vi "LoadTrafficLightsQueue with Exit.vi"(0 "Queue Ref in":refnum<queue>, 2 "Walk":bool) -> ()   [LabVIEW 2012]
doc: "Used to Enqueue the Walk Element when Walk button has been pressed. Uses a Queue Reference to efficiently read the address of Red State, Enqueues rest of elements and places Walk State at the front of the Queue.\nFor use alongside VI's that require the Exit Element."
uses:
  Controls/Traffic Light States (with Walk and Exit State).ctl
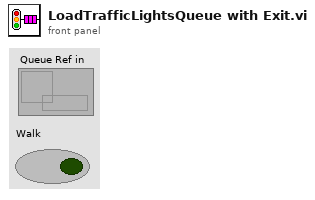
[diagram p1: front panel]
types:
  T1 = typedef "Traffic Light States (with Walk and Exit State).ctl" = enum16{"Red", "RedAmber", "Green", "Amber", "Walk", "Exit"}
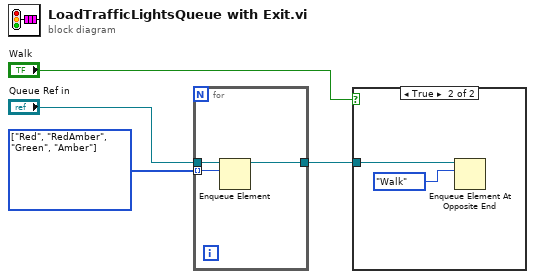
[diagram p0: block diagram]
diagram:
  w1 = T1[] [enum."Red", enum."RedAmber", enum."Green", enum."Amber"] items=["Red", "RedAmber", "Green", "Amber", "Walk", "Exit"]
  n1 = for {
    tunnel: "Queue Ref in" -> [w7]
    tunnel: [w6] -> w3
    tunnel: w1 -> [w5] mode=indexing
    n2 = Enqueue Element(queue=w7, element=w5) -> (queue out=w6:refnum<queue>)  [unwired: 2 in, 2 out]
  }
  n3 = case "Walk Tunnel\nWalk Tunnel" shown="True" "Walk" {
    tunnel: w3 -> [_ w9]
    frame False {
    }
    frame True {
      n4 = Enqueue Element At Opposite End(queue=w9, element=Traffic_Light_States_(with_Walk_and_Exit_State)."Walk") -> ()  [unwired: 2 in, 3 out]
    }
  }
